vi "RTD_R_to_temp.vi"(1 "RTD coefficients":dbl[](array[numeric])=[100.0, 0.00390802, -5.80195e-07], 2 "R [Ohm]":dbl, 4 "use inverse":bool, 5 "RTD inverse poly":dbl[](array[numeric])=[100.0, 0.00390802, -5.80195e-07]) -> (7 "t [deg C]":dbl)   [LabVIEW 2020]
uses:
  <vilib>/Utility/TradDaqScaling.llb/Convert RTD Reading (scaler).vi
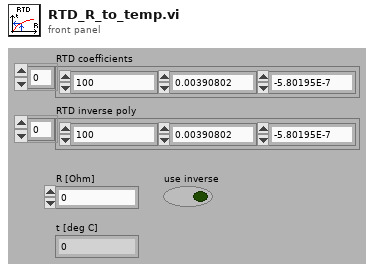
[diagram p1: front panel]
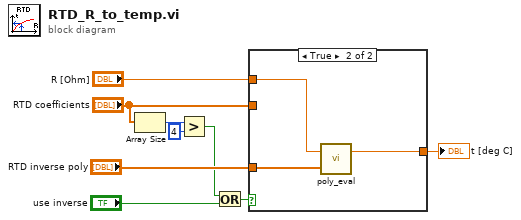
[diagram p0: block diagram]
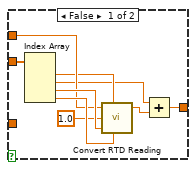
[diagram p2: hidden frame]
diagram:
  n1 = Array Size(array="RTD coefficients") -> (size(s)=w5:i32)
  n2 = Greater?(x=w5, y=4) -> (0:w2:bool)
  n3 = Or(x=w2, y="use inverse") -> (x .or. y?=w3:bool)
  n4 = case shown="True" w3 {
    tunnel: "R [Ohm]" -> [w15 w20]
    tunnel: [w11 w21] -> w8
    tunnel: "RTD coefficients" -> [w14 _]
    tunnel: "RTD inverse poly" -> [_ w19]
    frame False {
      n5 = Index Array(array=w14) -> (element #1=w13:dbl, element #2=w10:dbl, element #3=w18:dbl, element #4=w17:dbl)  [unwired: 4 in]
      n6 = call-poly <vilib>:"Convert RTD Reading.vi"("RTDvolts"=w15, "Ro"=w13, "Iex"=sgl 1.0, "A"=w18, "B"=w17) -> ("RTDtemp"=w12:sgl)  [unwired: 2 in]
      n7 = Add(x=w10, y=w12) -> (x+y=w11:dbl)
    }
    frame True {
      n8 = call "poly_eval.vi"("P(x)"=w19, "A"=w20) -> ("P(A)"=w21:dbl)  [unwired: 1 in]
    }
  }
  "t [deg C]" <- w8
